vi "get spotfield.vi"(8 "error in (no error)":errorcluster, 11 "VISA Refnum in":refnum<visa-resource-name>) -> (0 "error out":errorcluster, 1 "Boolean array":bool[](array[boolean]), 2 "ImageBuf":u8[][](array[numeric]), 3 "VISA Refnum out":refnum<visa-resource-name>, 4 "timedout":bool)   [LabVIEW 2020, in "ThorlabsWFS.lvclass"]
uses:
  ThorlabsWFS.lvclass
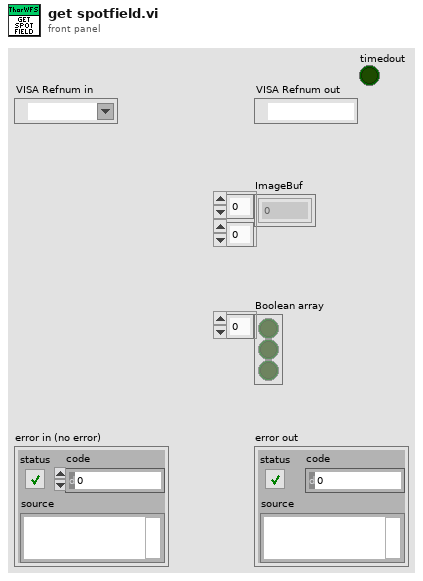
[diagram p1: front panel]
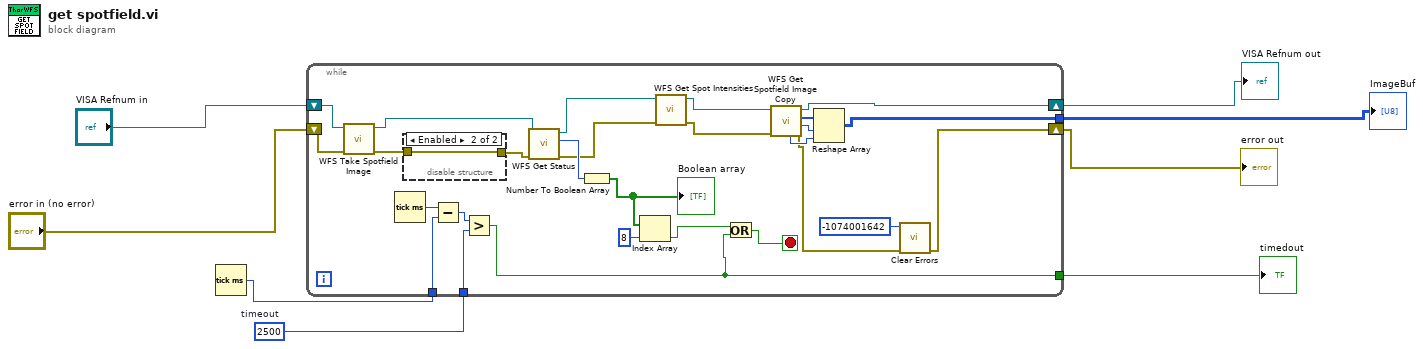
[diagram p0: block diagram]
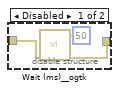
[diagram p2: hidden frame]
diagram:
  w1 = u32 2500  # timeout
  n1 = Tick Count (ms)() -> (millisecond timer value=w3:u32)
  n2 = while {
    shift-right: [w21] -> w4
    shift-left: "error in (no error)" -> [w34]
    shift-right: [w23] -> w5
    shift-left: "VISA Refnum in" -> [w33]
    tunnel: [w24] -> w6
    tunnel: w3 -> [w14]
    tunnel: w1 -> [w12]
    tunnel: [w9] -> w2
    stop <- w10 stop-if-true
    n3 = call "WFS Take Spotfield Image.vi"("error in (no error)"=w34, "instrument handle"=w33) -> ("error out"=w31:errorcluster, "instrument handle out"=w35:refnum<visa-resource-name>)  [unwired: 8 in]
    n4 = Tick Count (ms)() -> (millisecond timer value=w15:u32)
    n5 = disable-structure shown="Enabled" {
      disable-tunnel: [w38 w39] -> w32
      disable-tunnel: w31 -> [w37 w39]
      frame Disabled {
        n6 = call "Wait (ms)__ogtk.vi"("error in (no error)"=w37, "milliseconds to wait"=u32 50) -> ("error out"=w38:errorcluster)  [unwired: 8 in, 1 out]
      }
      frame Enabled {
      }
    }
    n7 = Subtract(x=w15, y=w14) -> (x-y=w13:u32)
    n8 = Greater?(x=w13, y=w12) -> (0:w9:bool)
    n9 = call "WFS Get Status.vi"("error in (no error)"=w32, "instrument handle"=w35) -> ("error out"=w17:errorcluster, "Device Status"=w30:i32, "instrument handle out"=w19:refnum<visa-resource-name>)  [unwired: 7 in]
    n10 = Number To Boolean Array(number=w30) -> (Boolean array=w29:bool[])
    "Boolean array" <- w29
    n11 = Index Array(array=w29, index=8) -> (element=w11:bool)
    n12 = call "WFS Get Spot Intensities.vi"("error in (no error)"=w17, "instrument handle"=w19) -> ("error out"=w16:errorcluster, "instrument handle out"=w18:refnum<visa-resource-name>)  [unwired: 7 in, 1 out]
    n13 = Or(x=w11, y=w9) -> (x .or. y?=w10:bool)
    n14 = call "WFS Get Spotfield Image Copy.vi"("error in (no error)"=w16, "instrument handle"=w18) -> ("error out"=w22:errorcluster, "Rows"=w27:i32, "ImageBuf"=w25:u8[], "instrument handle out"=w23:refnum<visa-resource-name>, "Columns"=w26:i32)  [unwired: 5 in]
    n15 = Reshape Array(w25, w27, w26) -> (w24:u8[][])
    n16 = call "Clear Errors.vi"("error in (no error)"=w22, "specific error code to clear (0: all)"=-1074001642) -> ("error out"=w21:errorcluster)  [unwired: 4 in, 1 out]
  }
  "error out" <- w4
  "VISA Refnum out" <- w5
  "ImageBuf" <- w6
  "timedout" <- w2
